vi "GenBreathe.vi"(6 "Reset":bool, 9 "Sine Rate":i32=30, 10 "Color Box":u32(colorbox)=16711680, 11 "NumLeds":i32) -> (2 "Iterator":i32, 3 "Array":u32[](array[numeric]))   [LabVIEW 2023, in "ArduinoSerialBling.lvlib"]
uses:
  ArduinoSerialBling.lvlib
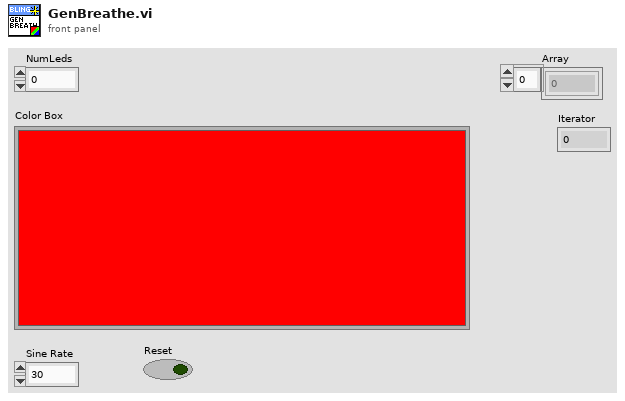
[diagram p1: front panel]
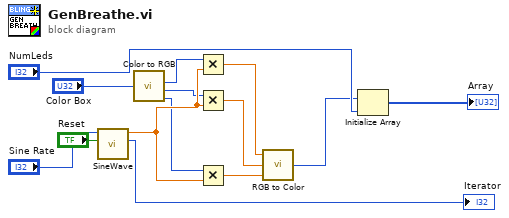
[diagram p0: block diagram]
diagram:
  n1 = call "SineWave.vi"("Reset"="Reset", "Sine Rate"="Sine Rate") -> ("Iterator"=→"Iterator":i32, "Value (0-1)"=w13:dbl)  [unwired: 8 in]
  n2 = call <vilib>:"Color to RGB.vi"("Color"="Color Box") -> ("R"=w9:u8, "G"=w10:u8, "B"=w11:u8)  [unwired: 1 out]
  n3 = Multiply(x=w9, y=w13) -> (x*y=w4:dbl)
  n4 = Multiply(x=w10, y=w13) -> (x*y=w5:dbl)
  n5 = Multiply(x=w11, y=w13) -> (x*y=w6:dbl)
  n6 = call <vilib>:"RGB to Color.vi"("B"=w6, "G"=w5, "R"=w4) -> ("Color"=w7:u32)
  n7 = Initialize Array(w7, "NumLeds") -> (→"Array":u32[])
